vi "Create Plot Object.vi"(6 "Control Ref Queue":T1, 7 "Actual Transform In":T2, 8 "error in (no error)":errorcluster, 9 "Multiplot Representation In":T4, 10 "3D Pie.lvclass in":refnum<class "3D Pie.lvclass">, 11 "Plot Object In":refnum<vi>) -> (0 "error out":errorcluster, 1 "Multiplot Representation Out":T4, 2 "3D Pie.lvclass out":refnum<class "3D Pie.lvclass">, 3 "Plot Object Out":refnum<vi>, 5 "Actual Transform Out":T2)   [LabVIEW 2020, in "3D Pie.lvclass"]
uses:
  <vilib>/Math Plots/3D Math Plots/3D Pie/3D Pie/3D Pie.lvclass
  <vilib>/Math Plots/3D Math Plots/3D Plot/3D Plot/Typedef/Multiplot Representation.ctl
  <vilib>/Math Plots/3D Math Plots/3D Plot/3D Plot/Typedef/Plot Representation.ctl
  <vilib>/Math Plots/3D Math Plots/3D Plot/3D Plot/Typedef/Range Clusters.ctl
  <vilib>/Math Plots/3D Math Plots/3D Plot/3D Plot/Typedef/Mesh Data.ctl
  <vilib>/Math Plots/3D Math Plots/3D Plot/3D Plot/Typedef/Actual Transform.ctl
  <vilib>/Math Plots/3D Math Plots/3D Plot/Action String/3DMathPlot Ctrl Act Queue.ctl
  <vilib>/Math Plots/3D Math Plots/3D Plot/Action String/3DMathPlot Ctrl Act Cluster.ctl
  <vilib>/Math Plots/3D Math Plots/3D Plot/Action String/3DMathPlot State Class.ctl
  <vilib>/Math Plots/3D Math Plots/3D Pie/3D Pie/3D Pie.lvclass/3D Pie.ctl
  <vilib>/Math Plots/3D Math Plots/3D Plot/3D Plot/3D Plot.lvclass
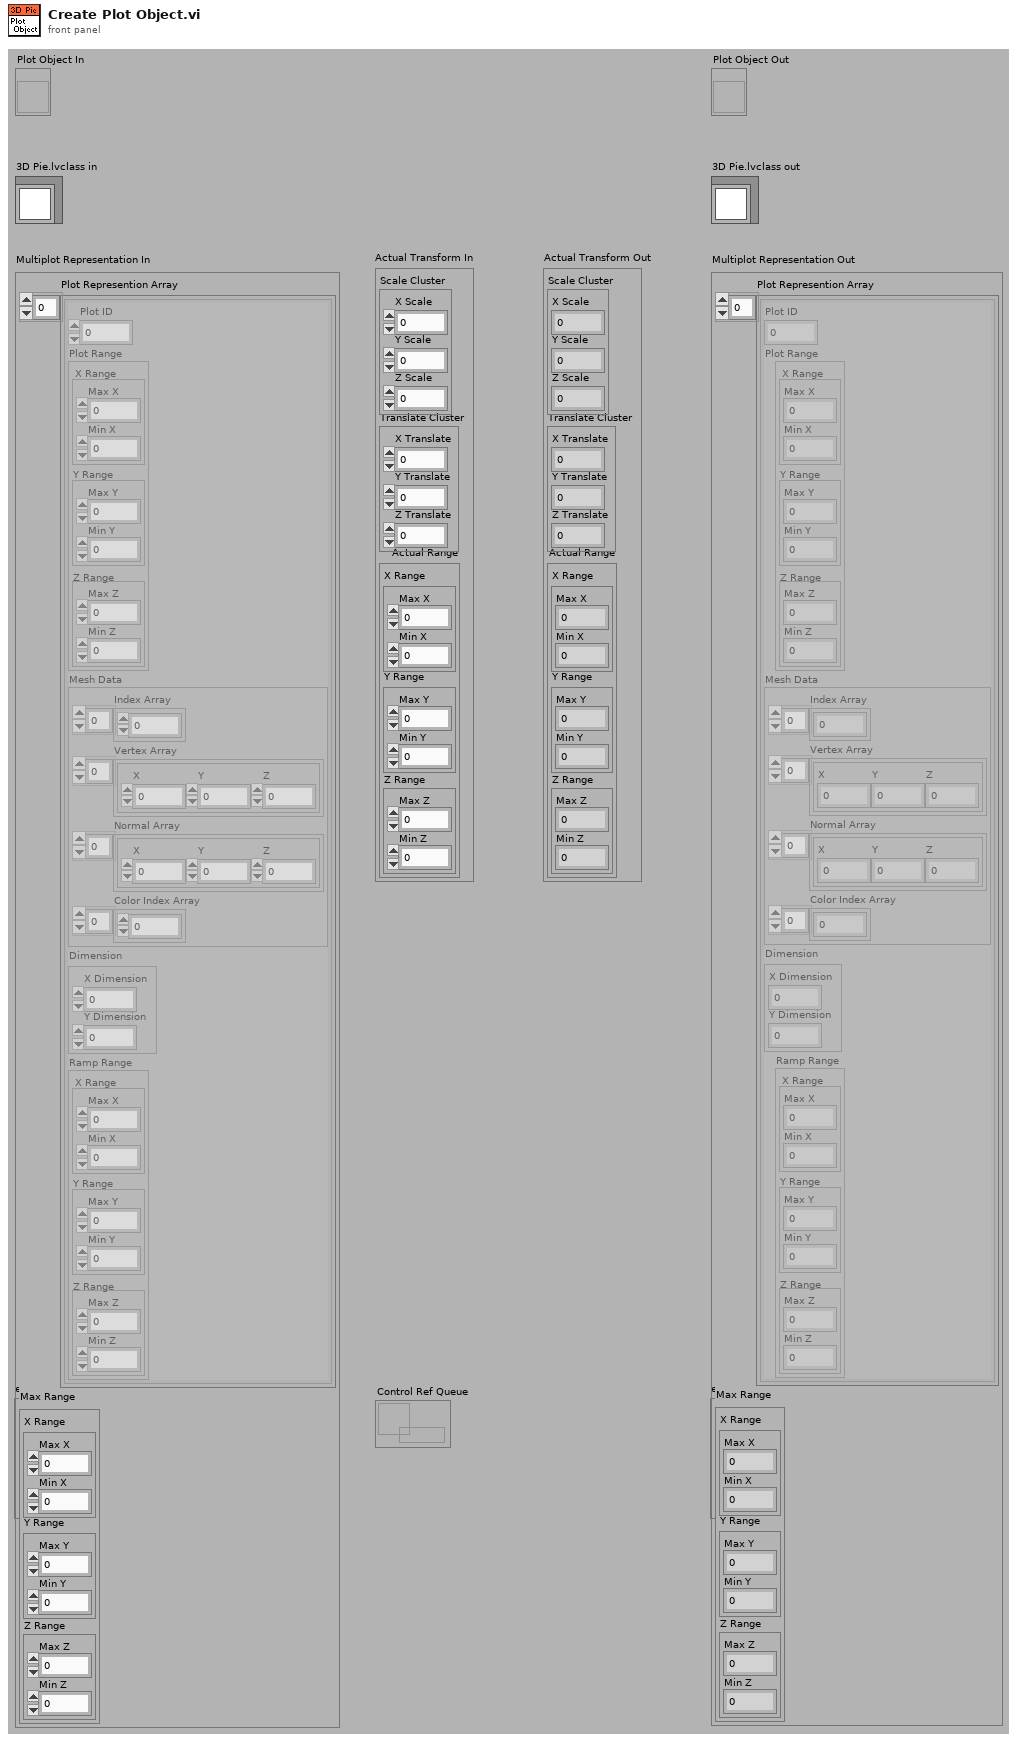
[diagram p1: front panel]
types:
  T1 = typedef "3DMathPlot Ctrl Act Queue.ctl" = refnum<queue>
  T2 = typedef "3D Plot.lvclass/Actual Transform.ctl" = cluster{"Scale Cluster":cluster{"X Scale":sgl, "Y Scale":sgl, "Z Scale":sgl}, "Translate Cluster":cluster{"X Translate":sgl, "Y Translate":sgl, "Z Translate":sgl}, "Actual Range":T3}
  T3 = typedef "3D Plot.lvclass/Range Clusters.ctl" = cluster{"X Range":cluster{"Max X":sgl, "Min X":sgl}, "Y Range":cluster{"Max Y":sgl, "Min Y":sgl}, "Z Range":cluster{"Max Z":sgl, "Min Z":sgl}}
  T4 = typedef "3D Plot.lvclass/Multiplot Representation.ctl" = cluster{"Plot Represention Array":T5[], "Max Range":T3}
  T5 = typedef "3D Plot.lvclass/Plot Representation.ctl" = cluster{"Plot ID":i32, "Plot Range":T3, "Mesh Data":T6, "Dimension":cluster{"X Dimension":i32, "Y Dimension":i32}, "Ramp Range":T3}
  T6 = typedef "3D Plot.lvclass/Mesh Data.ctl" = cluster{"Index Array":u32[], "Vertex Array":cluster{"X":sgl, "Y":sgl, "Z":sgl}[], "Normal Array":cluster{"X":sgl, "Y":sgl, "Z":sgl}[], "Color Index Array":i32[]}
  T7 = typedef "3D Pie.lvclass/3D Pie Property Array.ctl" = T8[]
  T8 = typedef "3D Pie.lvclass/3D Pie Property.ctl" = cluster{"General Property":cluster{"Plot Name":string, "Coordinate System":enum16{"Cartesian", "Cylindrical", "Spherical"}, "Opacity":sgl}, "Projection Property":cluster{"Draw XY":bool, "Draw YZ":bool, "Draw XZ":bool}, "Plot Property":cluster{"Line Style":T9, "Line Width":sgl, "Line Color":u32, "Antialiasing":bool}, "Pie Property":cluster{"Pie Height":sgl, "Pie Center":cluster{"X":sgl, "Y":sgl, "Z":sgl}, "Label Mode":enum16{"None", "Show Percentage", "Show String"}, "Label Size":u16, "Label Color":u32, "Color Pair Array":cluster{"Color":u32, "String":string}[], "Slice Offset?":bool}}
  T9 = typedef "3D Plot.lvclass/Line Type.ctl" = enum16{"None", "Solid", "Dash", "Dot", "Dash Dot"}
  T10 = enum16{"Points", "Lines", "Line Strip", "Line Loop", "Triangles", "Triangle Strip", "Triangle Fan", "Quads", "Quad Strip", "Polygon"}
  T11 = cluster{"Draw XY":bool, "Draw YZ":bool, "Draw XZ":bool}
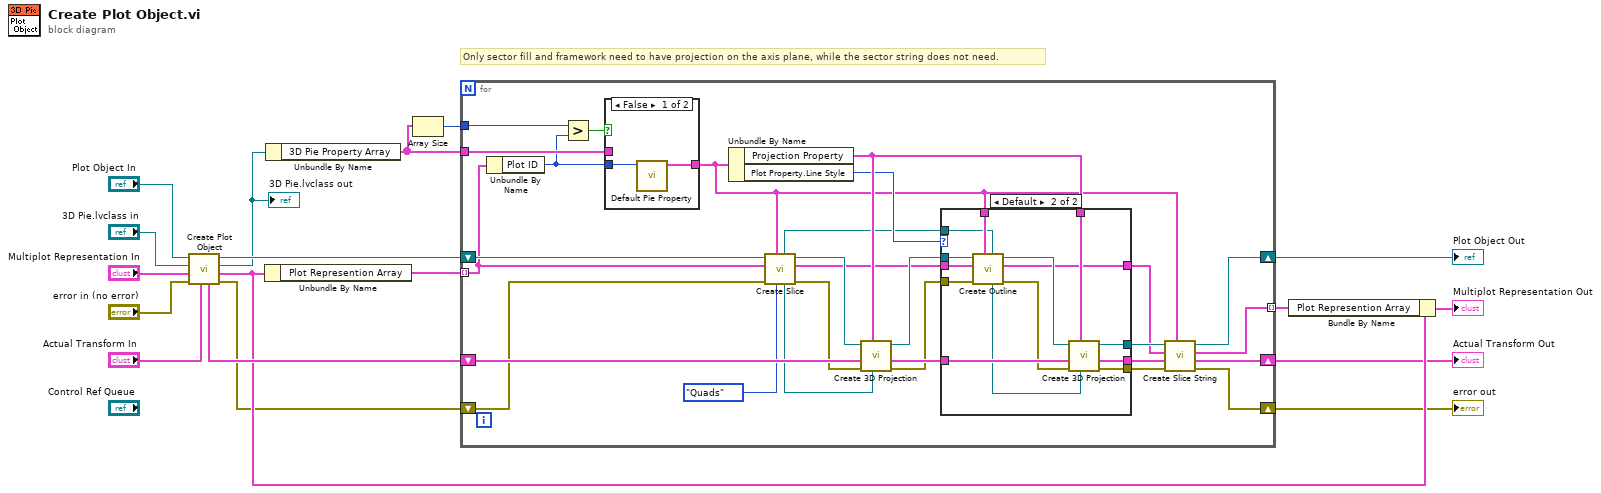
[diagram p0: block diagram]
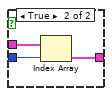
[diagram p2: hidden frame]
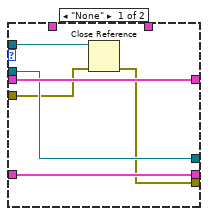
[diagram p3: hidden frame]
diagram:
  # "Only sector fill and framework need to have projection on the axis plane, while the sector string does not need."
  n1 = call-parent "Create Plot Object.vi"("Actual Transform In"="Actual Transform In", "error in (no error)"="error in (no error)", "Multiplot Representation In"="Multiplot Representation In", "3D Plot.lvclass in"="3D Pie.lvclass in", "Plot Object In"="Plot Object In") -> ("error out"=w3:errorcluster, "Multiplot Representation Out"=w10:T4, "3D Plot.lvclass out"=w4:refnum<class "3D Pie.lvclass">, "Plot Object Out"=w6:refnum<vi>, "Actual Transform Out"=w11:T2)  [unwired: 1 in, 1 out]
  "3D Pie.lvclass out" <- w4
  n2 = Unbundle By Name(w10) -> ("Plot Represention Array"=w13:T5[])
  n3 = Unbundle By Name(w4) -> ("3D Pie Property Array"=w1:T7)
  n4 = Array Size(array=w1) -> (size(s)=w2:i32)
  n5 = for {
    tunnel: [w45] -> w12 mode=indexing
    shift-right: [w46] -> w5
    shift-left: w6 -> [w36]
    shift-right: [w43] -> w7
    shift-left: w3 -> [w33]
    shift-right: [w44] -> w8
    shift-left: w11 -> [w42]
    tunnel: w13 -> [w34] mode=indexing
    tunnel: w1 -> [w23]
    tunnel: w2 -> [w21]
    n6 = Unbundle By Name(w34) -> ("Plot ID"=w22:i32)
    n7 = Greater?(x=w21, y=w22) -> (0:w24:bool)
    n8 = case shown="False" w24 {
      tunnel: w23 -> [_ w51]
      tunnel: [w47 w50] -> w20
      tunnel: w22 -> [w48 w49]
      frame False {
        n9 = call <vilib>:"Default Pie Property.vi"("Plot ID"=w48) -> ("Default Property"=w47:T8)  [unwired: 10 out]
      }
      frame True {
        n10 = Index Array(array=w51, index=w49) -> (element=w50:T8)
      }
    }
    n11 = Unbundle By Name(w20) -> ("Projection Property"=w37:T11, "Plot Property.Line Style"=w25:T9)
    n12 = call <vilib>:"Create Slice.vi"("Draw Mode"=T10."Quads", "3D Pie Property"=w20, "error in (no error)"=w33, "Plot Representation In"=w34, "Plot Object In"=w36) -> ("error out"=w32:errorcluster, "Plot Representation Out"=w30:T5, "Plot Object Out"=w35:refnum<vi>, "Sector Object Out"=w26:refnum<vi>, "Drawable"=w19:refnum<vi>)  [unwired: 2 out]
    n13 = call <vilib>:"Create 3D Projection.vi"("Sub Object In"=w26, "Projection Property"=w37, "error in (no error)"=w32, "Actual Transform In"=w42, "Plot Object In"=w35) -> ("error out"=w29:errorcluster, "Actual Transform Out"=w39:T2, "Plot Object Out"=w31:refnum<vi>)  [unwired: 1 in, 3 out]
    n14 = case shown="Default" w25 {
      tunnel: [w56 w71] -> w41
      tunnel: [w55 w70] -> w40
      tunnel: w39 -> [w55 w69]
      tunnel: [w53 w68] -> w38
      tunnel: w37 -> [_ w67]
      tunnel: w31 -> [w56 w65]
      tunnel: w30 -> [w57 w64]
      tunnel: w29 -> [w54 w63]
      tunnel: [w57 w61] -> w28
      tunnel: w20 -> [_ w60]
      tunnel: w19 -> [w52 w58]
      frame "None" {
        n15 = Close Reference(reference=w52, error in (no error)=w54) -> (error out=w53:errorcluster)
      }
      frame Default {
        n16 = call <vilib>:"Create Outline.vi"("Drawable"=w58, "3D Pie Property"=w60, "error in (no error)"=w63, "Plot Representation In"=w64, "Plot Object In"=w65) -> ("error out"=w62:errorcluster, "Plot Representation Out"=w61:T5, "Plot Object Out"=w66:refnum<vi>, "Outline Object Out"=w59:refnum<vi>)  [unwired: 3 out]
        n17 = call <vilib>:"Create 3D Projection.vi"("Sub Object In"=w59, "Projection Property"=w67, "error in (no error)"=w62, "Actual Transform In"=w69, "Plot Object In"=w66) -> ("error out"=w68:errorcluster, "Actual Transform Out"=w70:T2, "Plot Object Out"=w71:refnum<vi>)  [unwired: 1 in, 3 out]
      }
    }
    n18 = call <vilib>:"Create Slice String.vi"("3D Pie Property"=w20, "error in (no error)"=w38, "Actual Transform In"=w40, "Plot Representation In"=w28, "Plot Object In"=w41) -> ("error out"=w43:errorcluster, "Actual Transform Out"=w44:T2, "Plot Representation Out"=w45:T5, "Plot Object Out"=w46:refnum<vi>)  [unwired: 1 in, 2 out]
  }
  "error out" <- w7
  "Plot Object Out" <- w5
  "Actual Transform Out" <- w8
  n19 = Bundle By Name(cluster=w10, "Plot Represention Array"=w12) -> (→"Multiplot Representation Out":T4)
